vi "Write_Data.vi"(4 "error in":errorcluster, 5 "Data cluster in":cluster{dbl[], dbl[]}, 6 "Header":string, 7 "file path":path) -> (0 "error out":errorcluster)   [LabVIEW 2022 SP3]
panel:
  # "Voltage"
  # "Current"
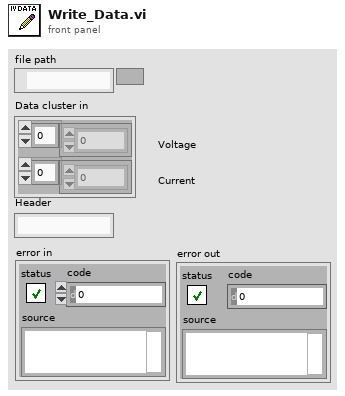
[diagram p1: front panel]
types:
  T1 = enum16{"open", "replace", "create", "open or create", "replace or create", "replace or create with confirmation"}
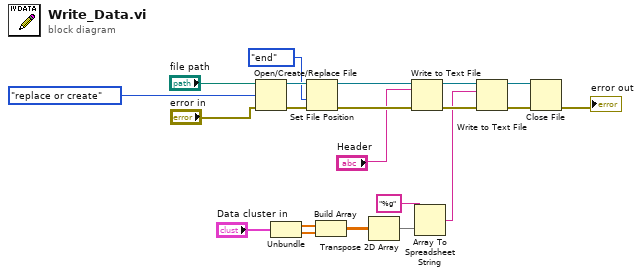
[diagram p0: block diagram]
diagram:
  n1 = Open/Create/Replace File(file path (use dialog)="file path", error in="error in", operation (0:open)=T1."replace or create") -> (refnum out=w13:refnum<file>, error out=w12:errorcluster)  [unwired: 3 in, 1 out]
  n2 = Unbundle("Data cluster in") -> (w20:dbl[], w19:dbl[])
  n3 = Set File Position(refnum=w13, from (0:start)=enum16{"start", "end", "current"}."end", error in=w12) -> (refnum out=w10:refnum<file>, error out=w11:errorcluster)  [unwired: 1 in]
  n4 = Build Array(w20, w19) -> (w18:dbl[][])
  n5 = Transpose 2D Array(2D array=w18) -> (transposed array=w17:dbl[][])
  n6 = Write to Text File(file (use dialog)=w10, text="Header", error in=w11) -> (refnum out=w16:refnum<file>, error out=w15:errorcluster)  [unwired: 1 in, 1 out]
  n7 = Array To Spreadsheet String(array=w17, 3:"%g" ("format string")) -> (spreadsheet string=w14:string)  [unwired: 1 in]
  n8 = Write to Text File(file (use dialog)=w16, text=w14, error in=w15) -> (refnum out=w5:refnum<file>, error out=w4:errorcluster)  [unwired: 1 in, 1 out]
  n9 = Close File(refnum=w5, error in=w4) -> (error out=→"error out":errorcluster)  [unwired: 1 out]
